vi "Get Sample.vi"(1 "Waveform":waveform(dbl)) -> (0 "As scalar":dbl)   [LabVIEW 2021, in "Acquisition.lvlib"]
uses:
  Acquisition.lvlib
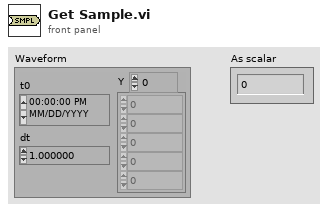
[diagram p1: front panel]
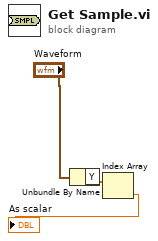
[diagram p0: block diagram]
diagram:
  n1 = Unbundle By Name("Waveform") -> ("Y"=w2:dbl[])
  n2 = Index Array(array=w2) -> (element=→"As scalar":dbl)  [unwired: 1 in]
